vi "TEST_r_w_L1_COMPLETE.vi"() -> ()   [LabVIEW 2012]
uses:
  <vilib>/Utility/NIReport.llb/NI_report.lvclass
  <vilib>/Utility/NIReport.llb/HTML/NI_HTML.lvclass
  Sum_Abrilader/L0_Sum_Adder Folder/C/Program Files/National Instruments/LabVIEW 2012/instr.lib/Agilent 8000 Series/Public/Configure/Configure Math (Binary Operation).vi
  Sum_Abrilader/L0_Sum_Adder Folder/C/Program Files/National Instruments/LabVIEW 2012/instr.lib/Agilent 8000 Series/Public/Data/Low Level/Fetch Measurement (More).vi
  Sum_Abrilader/L0_Sum_Adder Folder/C/Program Files/National Instruments/LabVIEW 2012/instr.lib/Agilent 8000 Series/Agilent 8000 Series.lvlib
panel:
  out "Measurement 2":dbl
  out "x*y":i32=65792
  out "Measurement":dbl=4350.000326699999
  out "data out serial":string="empty_read_bufferwrittingempty_read_bufferwritting2"
  in  "Instrument VISA in":T1={"AWG VISA"="AgilentGenerator1", "Oscilloscope  VISA "="AgilentOsciloscope", "Integration Board IP"="172.16.17.48", "connection ID"=refnum, "report out"=refnum, "report file path"=path "C:/Documents and Settings/CTA_LAB01/Desktop/L0_Asic/L0 Asic Test Data"}
  in  "Combination\n  (Act High)":i32=127 min=0 max=127 step=1 format="%b"
  in  "Single/Comb":bool
  in  "Single Channel Enable":i32(slide) scale=0.0..6.0
  out "error out":errorcluster
  in  "error in (no error)":errorcluster
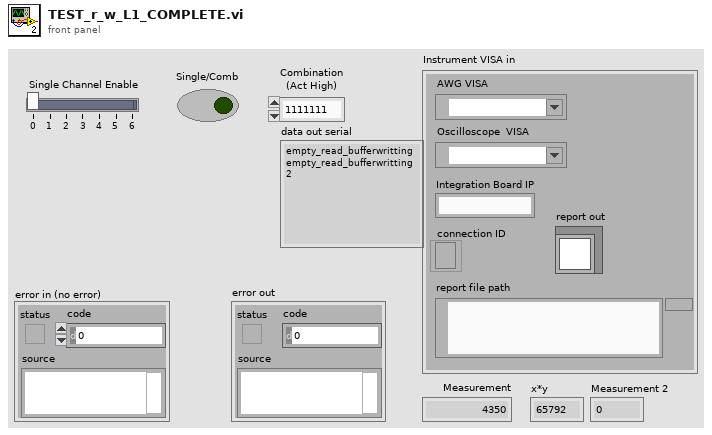
[diagram p1: front panel]
types:
  T1 = cluster{"AWG VISA":refnum<visa-resource-name>, "Oscilloscope  VISA ":refnum<visa-resource-name>, "Integration Board IP":string, "connection ID":refnum<k5>, "report out":refnum<class "NI_report.lvclass">, "report file path":path}
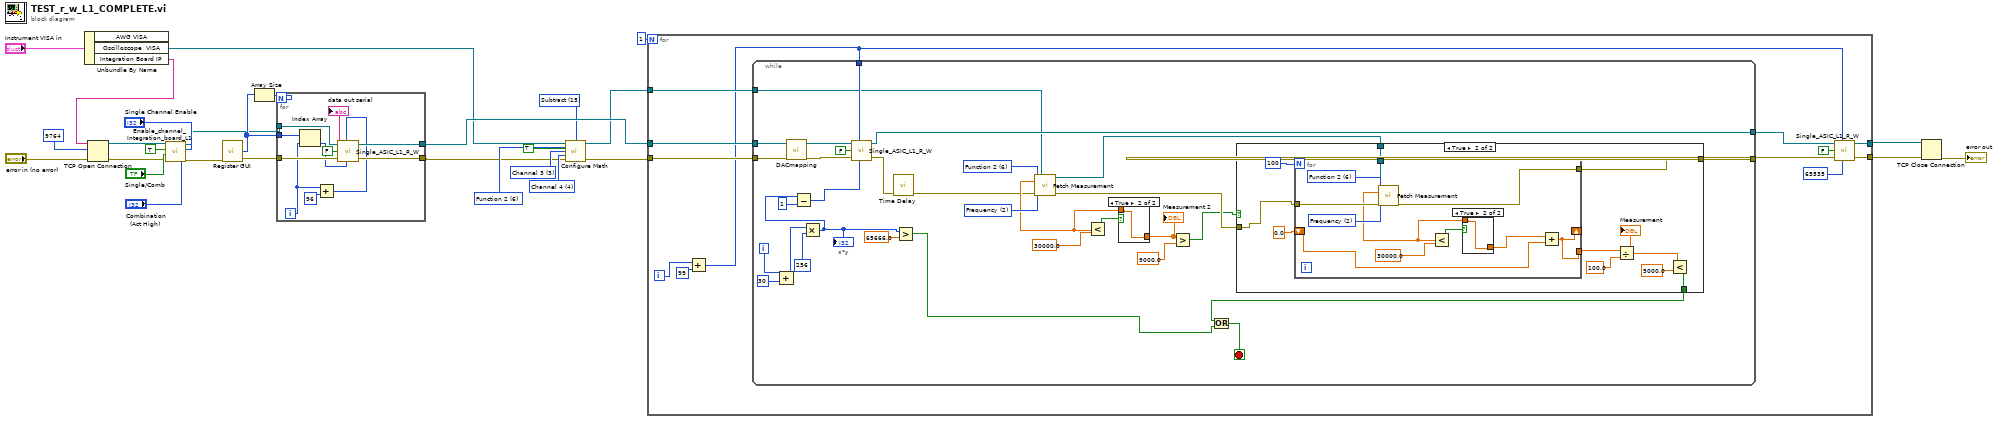
[diagram p0: block diagram]
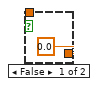
[diagram p2: hidden frame]
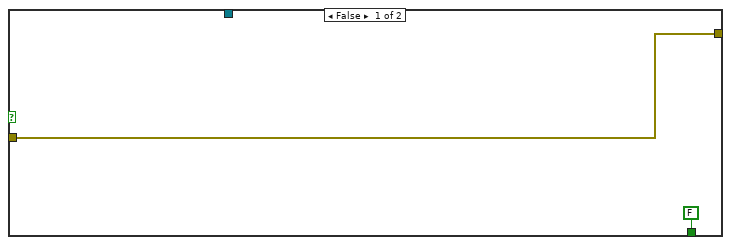
[diagram p3: hidden frame]
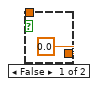
[diagram p4: hidden frame]
diagram:
  w5 = u16 6 items=["Function 1"=5, "Function 2"=6, "Function 3"=7, "Function 4"=8] ("Math Channel (5: Function 1)")
  w6 = u16 15 items=["Add"=12, "Divide"=13, "Multiply"=14, "Subtract"=15, "Common Mode"=16, "Versus"=17] ("Math Operation (12: Add)")
  w8 = 3 items=["Channel 1"=1, "Channel 2"=2, "Channel 3"=3, "Channel 4"=4] ("Channel (1: Channel 1)")
  w7 = 4 items=["Channel 1"=1, "Channel 2"=2, "Channel 3"=3, "Channel 4"=4] ("Channel (1: Channel 1)")
  n1 = Unbundle By Name("Instrument VISA in") -> ("Oscilloscope  VISA"=w3:refnum<visa-resource-name>, "Integration Board IP"=w11:string)  [unwired: 1 out]
  n2 = TCP Open Connection(address=w11, remote port or service name=9764, error in (no error)="error in (no error)") -> (connection ID=w21:refnum<k5>, error out=w22:errorcluster)  [unwired: 2 in]
  n3 = call "Enable_channel_Integration_board_L1.vi"("Cobination"="Combination\n  (Act High)", "Enable  L1 single  Input"="Single Channel Enable", "error in (no error)"=w22, "SingleIN/#Combination"="Single/Comb", "#Enable all L1"=TRUE, "connection ID"=w21) -> ("error out"=w12:errorcluster, "connection ID out"=w17:refnum<k5>)
  n4 = call "Register GUI.vi"("error in (no error)"=w12) -> ("error out"=w20:errorcluster, "REG ARRAy"=w18:u32[])  [unwired: 3 in]
  n5 = Array Size(array=w18) -> (size(s)=w19:i32)
  n6 = for {
    N: w19 -> [_]
    tunnel: w20 -> [w40]
    tunnel: w18 -> [w39]
    tunnel: w17 -> [w38]
    tunnel: [w37] -> w10
    tunnel: [w36] -> w4
    i -> [w32]
    n7 = Index Array(array=w39, index=w32) -> (element=w35:u32)
    n8 = Add(x=w32, y=96) -> (x+y=w33:i32)
    n9 = call "Single_ASIC_L1_R_W.vi"("connection ID"=w38, "Register or channel"=w33, "RD/#WR"=FALSE, "error in (no error)"=w40, "Data"=w35) -> ("data out serial"=→"data out serial":string, "connection ID out"=w37:refnum<k5>, "error out"=w36:errorcluster)  [unwired: 1 in, 1 out]
  }
  n10 = call-poly "Configure Math.vi"("VISA resource name"=w3, "Enable Math Channel (T:Enable)"=TRUE, "Math Operation (12: Add)"=w6, "Math Channel (5: Function 1)"=w5, "Math Operand (1: Channel 1)"=w8, "Math Operand (2: Channel 2)"=w7, "error in (no error)"=w4) -> ("VISA resource name out"=w2:refnum<visa-resource-name>, "error out"=w1:errorcluster)  [unwired: 7 in]
  n11 = for {
    N: 1 -> [_]
    tunnel: w10 -> [w52]
    tunnel: w1 -> [w49]
    tunnel: [w46] -> w15
    tunnel: w2 -> [w48]
    tunnel: [w44] -> w13
    i -> [w50]
    n12 = Add(x=w50, y=99) -> (x+y=w43:i32)
    n13 = while {
      tunnel: w52 -> [w83]
      tunnel: w43 -> [w81]
      tunnel: w49 -> [w80]
      tunnel: [w78] -> w47
      tunnel: w48 -> [w60]
      tunnel: [w75] -> w45
      i -> [w58]
      stop <- w71 stop-if-true
      w70 = 2 items=["Rise Time", "Fall Time", "Frequency", "Period", "Voltage RMS(AC)", "Voltage RMS(DC)", "Voltage RMS (AC,cycle)", "Voltage RMS (DC,cycle)", "Voltage Max", "Voltage Min", "Voltage Middle", "Voltage Vpp", "Voltage High", "Voltage Low", "Voltage Average", "Voltage Average (cycle)", "Width Negative", "Width Positive", "Duty Cycle Positive", "Amplitude", "Overshoot", "Preshoot", "Voltage Base", "Voltage Upper", "Time Max", "Time Min", "Color Grade Crossing", "Color Grade Eye Width", "Color Grade Eye Height", "Color Grade Eye Q-Factory", "Color Grade Eye Duty Cycle Distortion(Percent)", "Color Grade Eye Duty Cycle Distortion(Time)", "Color Grade Eye Jitter(PP)", "Color Grade Eye Width(RMS)", "Cycle-cycle Duty Jitter(Rising)", "Cycle-cycle Duty Jitter(Falling)", "Cycle-cycle Jitter(Rising)", "Cycle-cycle Jitter(Falling)", "Cycle-cycle - Width", "Cycle-cycle + Width", "Date Rate", "Unit Interval", "FFT Delta Frequency", "FFT Delta Magnitude", "FFT Frequency", "FFT Magnitude", "Slew Rate", "Area (Entire Display)", "Area(Single Cycle)", "Duty Cycle (Rising)", "Duty Cycle (Falling)"] ("Measurement Function (0: Rise Time)")
      w69 = 6 items=["Channel 1"=1, "Channel 2"=2, "Channel 3"=3, "Channel 4"=4, "Function 1"=5, "Function 2"=6, "Function 3"=7, "Function 4"=8, "Memory 1"=9, "Memory 2"=10, "Memory 3"=11, "Memory 4"=12] ("Channel (1: Channel 1)")
      n14 = Add(x=w58, y=30) -> (x+y=w57:i32)
      n15 = call "DACmapping.vi"("error in (no error)"=w80) -> ("error out"=w79:errorcluster)  [unwired: 9 in, 1 out]
      n16 = Multiply(x=w57, y=256) -> (x*y=w55:i32)
      "x*y" <- w55
      n17 = Subtract(x=w55, y=1) -> (x-y=w53:i32)
      n18 = call "Single_ASIC_L1_R_W.vi"("connection ID"=w83, "Register or channel"=w81, "RD/#WR"=FALSE, "error in (no error)"=w79, "Data"=w53) -> ("connection ID out"=w75:refnum<k5>, "error out"=w74:errorcluster)  [unwired: 1 in, 2 out]
      n19 = call "Time Delay"("error in (no error)"=w74) -> ("error out"=w65:errorcluster)  [unwired: 10 in]
      n20 = Greater?(x=w55, y=65666.0) -> (0:w73:bool)
      n21 = call-poly "Fetch Measurement.vi"("VISA resource name"=w60, "Channel (1: Channel 1)"=w69, "Measurement Function (0: Rise Time)"=w70, "error in (no error)"=w65) -> ("VISA resource name out"=w59:refnum<visa-resource-name>, "Measurement"=w67:dbl, "error out"=w64:errorcluster)  [unwired: 9 in]
      n22 = Less?(x=w67, y=30000.0) -> (x < y?=w66:bool)
      n23 = case shown="True" w66 {
        tunnel: w67 -> [_ w85]
        tunnel: [0.0 ("Measurement") w85] -> w63
        frame False {
        }
        frame True {
        }
      }
      "Measurement 2" <- w63
      n24 = Greater?(x=w63, y=9000.0) -> (0:w61:bool)
      n25 = case shown="True" w61 {
        tunnel: [w87 w97] -> w78
        tunnel: [FALSE w90] -> w72
        tunnel: w59 -> [_ w89]
        tunnel: w64 -> [w87 w88]
        frame False {
        }
        frame True {
          n26 = for {
            N: 100 -> [_]
            tunnel: [w106] -> w97
            tunnel: w89 -> [w105]
            tunnel: w88 -> [w104]
            tunnel: [w100] -> w94
            shift-right: [w100] -> _
            shift-left: 0.0 -> [w99]
            w108 = 2 items=["Rise Time", "Fall Time", "Frequency", "Period", "Voltage RMS(AC)", "Voltage RMS(DC)", "Voltage RMS (AC,cycle)", "Voltage RMS (DC,cycle)", "Voltage Max", "Voltage Min", "Voltage Middle", "Voltage Vpp", "Voltage High", "Voltage Low", "Voltage Average", "Voltage Average (cycle)", "Width Negative", "Width Positive", "Duty Cycle Positive", "Amplitude", "Overshoot", "Preshoot", "Voltage Base", "Voltage Upper", "Time Max", "Time Min", "Color Grade Crossing", "Color Grade Eye Width", "Color Grade Eye Height", "Color Grade Eye Q-Factory", "Color Grade Eye Duty Cycle Distortion(Percent)", "Color Grade Eye Duty Cycle Distortion(Time)", "Color Grade Eye Jitter(PP)", "Color Grade Eye Width(RMS)", "Cycle-cycle Duty Jitter(Rising)", "Cycle-cycle Duty Jitter(Falling)", "Cycle-cycle Jitter(Rising)", "Cycle-cycle Jitter(Falling)", "Cycle-cycle - Width", "Cycle-cycle + Width", "Date Rate", "Unit Interval", "FFT Delta Frequency", "FFT Delta Magnitude", "FFT Frequency", "FFT Magnitude", "Slew Rate", "Area (Entire Display)", "Area(Single Cycle)", "Duty Cycle (Rising)", "Duty Cycle (Falling)"] ("Measurement Function (0: Rise Time)")
            w107 = 6 items=["Channel 1"=1, "Channel 2"=2, "Channel 3"=3, "Channel 4"=4, "Function 1"=5, "Function 2"=6, "Function 3"=7, "Function 4"=8, "Memory 1"=9, "Memory 2"=10, "Memory 3"=11, "Memory 4"=12] ("Channel (1: Channel 1)")
            n27 = call-poly "Fetch Measurement.vi"("VISA resource name"=w105, "Channel (1: Channel 1)"=w107, "Measurement Function (0: Rise Time)"=w108, "error in (no error)"=w104) -> ("Measurement"=w102:dbl, "error out"=w106:errorcluster)  [unwired: 9 in, 1 out]
            n28 = Less?(x=w102, y=30000.0) -> (x < y?=w101:bool)
            n29 = case shown="True" w101 {
              tunnel: w102 -> [_ w110]
              tunnel: [0.0 ("Measurement") w110] -> w98
              frame False {
              }
              frame True {
              }
            }
            n30 = Add(x=w98, y=w99) -> (x+y=w100:dbl)
          }
          n31 = Divide(x=w94, y=100.0) -> (x/y=w92:dbl)
          "Measurement" <- w92
          n32 = Less?(x=w92, y=5000.0) -> (x < y?=w90:bool)
        }
      }
      n33 = Or(x=w72, y=w73) -> (x .or. y?=w71:bool)
    }
    n34 = call "Single_ASIC_L1_R_W.vi"("connection ID"=w45, "Register or channel"=w43, "RD/#WR"=FALSE, "error in (no error)"=w47, "Data"=u32 65535 ("COMB DEC")) -> ("connection ID out"=w44:refnum<k5>, "error out"=w46:errorcluster)  [unwired: 1 in, 2 out]
  }
  n35 = TCP Close Connection(connection ID=w13, error in (no error)=w15) -> (error out=→"error out":errorcluster)  [unwired: 1 in, 1 out]
